vi "Remove.vi"(8 "error in (no error)":errorcluster, 10 "Test to Remove":string, 11 "LUnit Test Suite In":refnum<class "LUnit Test Suite.lvclass">) -> (0 "error out":errorcluster, 3 "LUnit Test Suite Out":refnum<class "LUnit Test Suite.lvclass">)   [LabVIEW 2020, in "LUnit Test Suite.lvclass"]
doc: "Remove a test by name from the test suite."
uses:
  LUnit Test Suite.lvclass
  LUnit Test Suite.lvclass/LUnit Test Suite.ctl
  Runnable.lvclass
  C:/git/astemes-lunit/source/LUnit Test Suite.lvclass
  C:/git/astemes-lunit/source/Runnable.lvclass
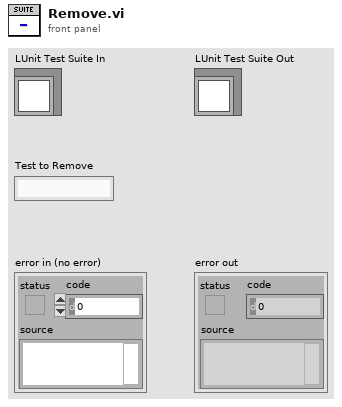
[diagram p1: front panel]
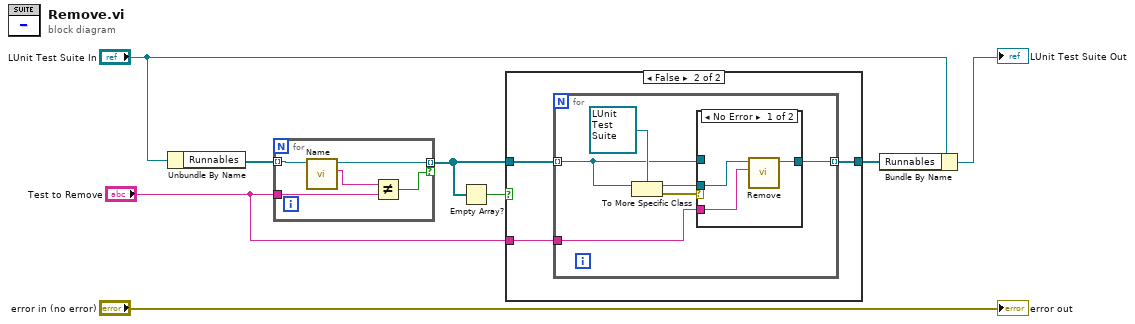
[diagram p0: block diagram]
diagram:
  n1 = Unbundle By Name("LUnit Test Suite In") -> ("Runnables"=w3:refnum<class "Runnable.lvclass">[])
  n2 = for {
    tunnel: w3 -> [w13] mode=indexing
    tunnel: [w12] -> w2 mode=indexing if=w9
    tunnel: "Test to Remove" -> [w10]
    n3 = call-dynamic "Name.vi"("Runnable in"=w13) -> ("Name"=w11:string, "Runnable out"=w12:refnum<class "Runnable.lvclass">)  [unwired: 8 in, 1 out]
    n4 = Not Equal?(x=w11, y=w10) -> (x != y?=w9:bool)
  }
  n5 = Empty Array?(array=w2) -> (empty?=w4:bool)
  n6 = case shown="False" w4 {
    tunnel: "Test to Remove" -> [_ w17]
    tunnel: [w14 w15] -> w5
    tunnel: w2 -> [w14 w16]
    frame True {
    }
    frame False {
      n7 = for {
        tunnel: w16 -> [w19] mode=indexing
        tunnel: w17 -> [w23]
        tunnel: [w18] -> w15 mode=indexing
        n8 = To More Specific Class(target class=refnum<class "LUnit Test Suite.lvclass"> refnum ("LUnit Test Suite.lvclass"), reference=w19) -> (specific class reference=w20:refnum<class "LUnit Test Suite.lvclass">, error out=w21:errorcluster)  [unwired: 1 in]
        n9 = case shown="No Error" w21 {
          tunnel: w20 -> [w26 _]
          tunnel: w23 -> [w25 _]
          tunnel: [w24 w27] -> w18
          tunnel: w19 -> [_ w27]
          frame No Error {
            n10 = call "Remove.vi"("Test to Remove"=w25, "LUnit Test Suite In"=w26) -> ("LUnit Test Suite Out"=w24:refnum<class "LUnit Test Suite.lvclass">)  [unwired: 8 in, 1 out]
          }
          frame Error {
          }
        }
      }
    }
  }
  n11 = Bundle By Name(cluster="LUnit Test Suite In", "Runnables"=w5) -> (→"LUnit Test Suite Out":refnum<class "LUnit Test Suite.lvclass">)
  "error out" <- "error in (no error)"
